vi "TAT_Varient Creater.vi"(8 "error in (no error)":errorcluster) -> (0 "error out":errorcluster)   [LabVIEW 2017]
uses:
  <vilib>/Utility/miscctls.llb/LVRangeTypeDef.ctl
  <vilib>/addons/database/Connection.llb/Conn ObjectReference.ctl
  <vilib>/Utility/miscctls.llb/LVRowAndColumnUnsignedTypeDef.ctl
  b1939813-2d0c-4b6e-8ee7-2e1edd5edc28.vi
  <vilib>/Utility/config.llb/Read Key (I32).vi
  <vilib>/Utility/config.llb/Read Key (String).vi
  <vilib>/Utility/config.llb/Write Key (U32).vi
  <vilib>/Utility/config.llb/Write Key (String).vi
  <vilib>/Utility/config.llb/NI_LVConfig.lvlib
  <vilib>/addons/database/NI_Database_API.lvlib
panel:
  in  "Vertical Slider Control":dbl(slide)=1.0
  in  "CANCLE 3":bool
  in  "PRINTING":bool
  in  "Manual print":bool
  in  "Cancle 2":bool
  in  "Delete Button":bool
  in  "Cancle":bool
  in  "Save Button":bool
  in  "TORISHI CODE":string
  in  "PART NUMBER":string
  in  "Delete Square":bool
  in  "EDIT & SAVE":bool
  out "Varient Details":string[][](table)
  in  "BATCH SIZE":u16=1 min=1 max=100 step=1
  in  "VARIENT NUMBER":u16=1 min=1 max=100 step=1
  in  "HOME":bool
  in  "UPDATE TABLE":bool
  in  "PART NAME":string(combo)
  # "Varient Creater"
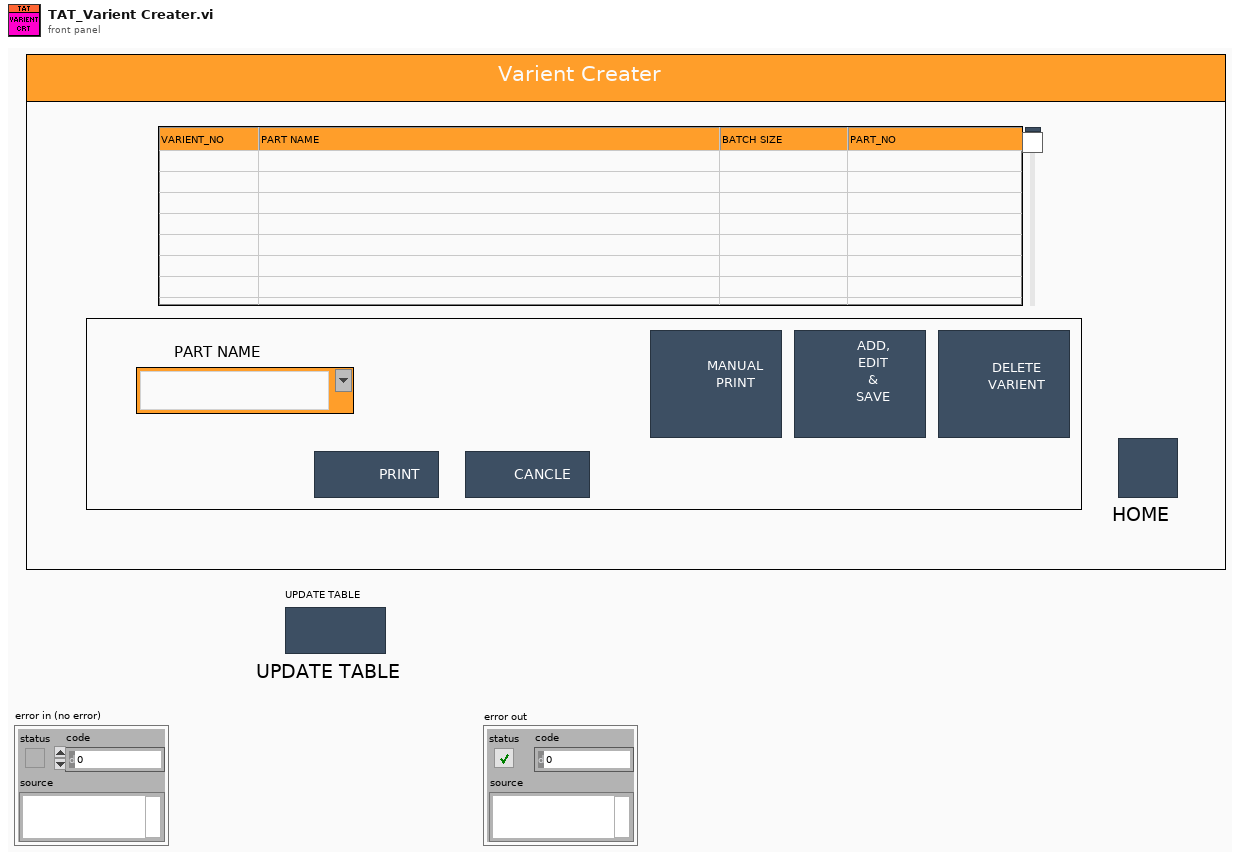
[diagram p1: front panel]
types:
  T1 = enum8{"Enabled", "Disabled", "Disabled and Grayed Out"}
  T2 = enum32{"invalid app kind", "Development System", "Run Time System", "Student Edition", "Embedded LabVIEW", "Evaluation", "Custom"}
  T3 = typedef "NI_LVConfig.lvlib/Config Data RefNum.ctl" = refnum<k1>
  T4 = typedef "LVRangeTypeDef.ctl" = cluster{"Minimum":dbl, "Maximum":dbl, "Increment":dbl, "Minor Increment":dbl, "Start":dbl}
  T5 = typedef "NI_Database_API.lvlib/Conn ObjectReference.ctl" = refnum<k1>
  T6 = cluster{"Varient number":u16, "Part name":string, "Barcode":string, "connection reference":T5, "Batch_Size":u16, "PART_NO":string, "TORISHI_CODE":string, "scanner com":refnum<visa-resource-name>, "Part Name List":string[], "Varient path":path, "Current Varient path":path, "Communication path":path, "PRN path":path, "printer":refnum<k5>, "Data_log_Path":path, "PREVIOUS Code":string[], "printer ip add":string}
  T7 = typedef "LVRowAndColumnUnsignedTypeDef.ctl" = cluster{"Row":u32, "Column":u32}
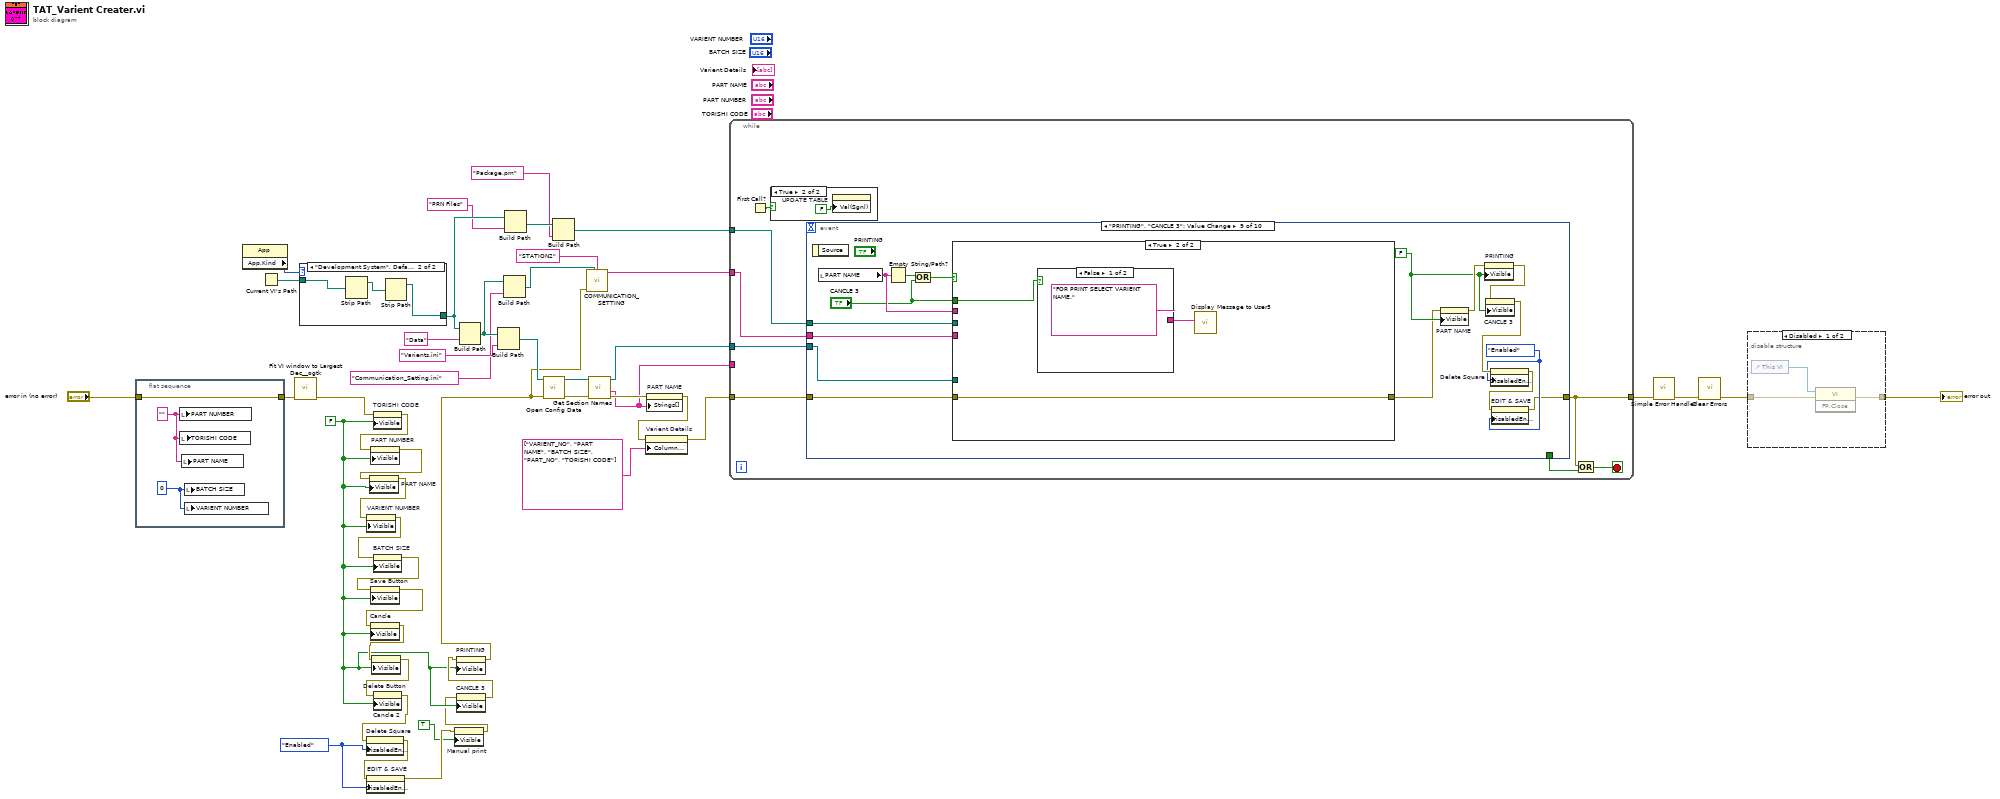
[diagram p0: block diagram]
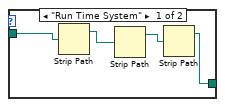
[diagram p3: hidden frame]
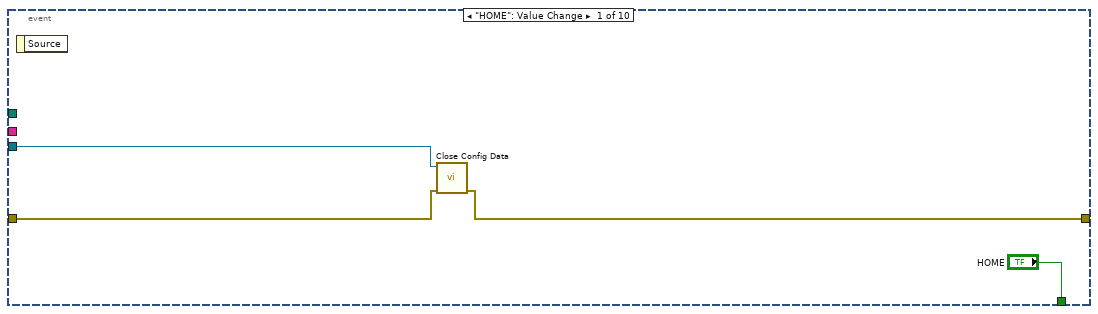
[diagram p5: hidden frame]
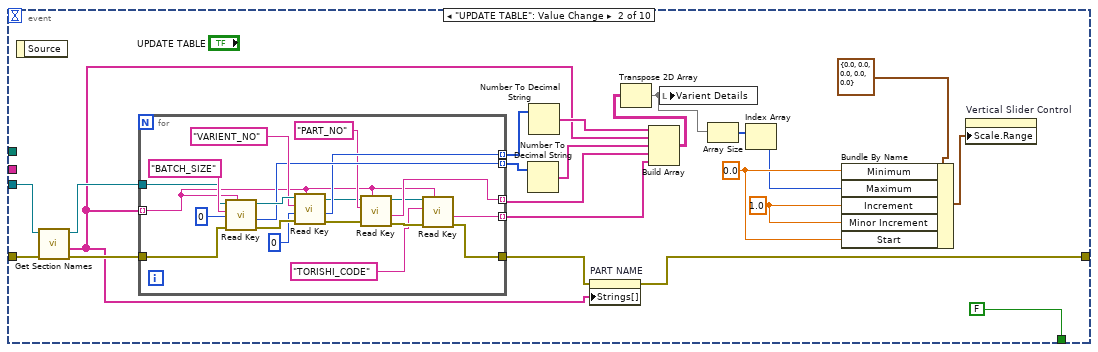
[diagram p6: hidden frame]
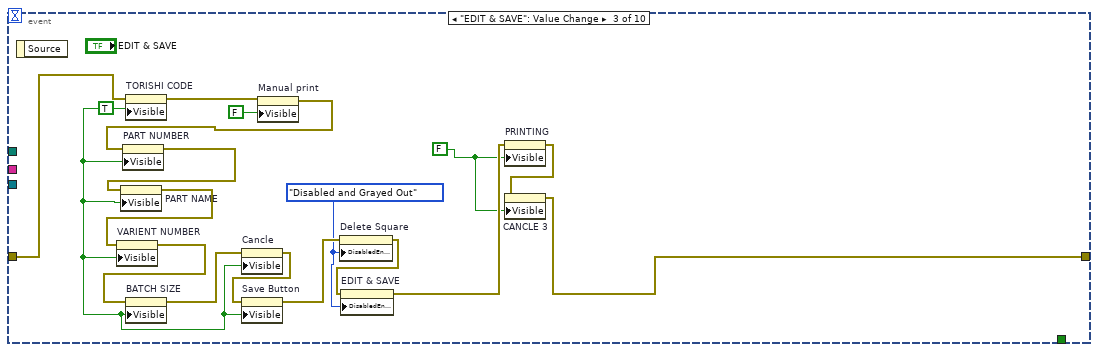
[diagram p7: hidden frame]
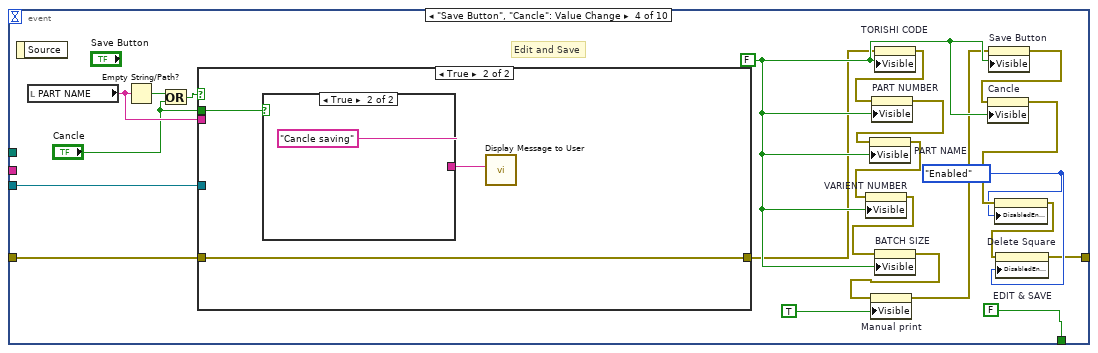
[diagram p8: hidden frame]
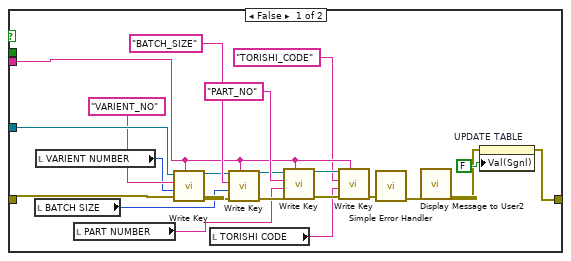
[diagram p9: hidden frame]
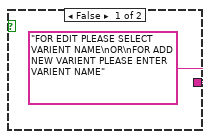
[diagram p10: hidden frame]
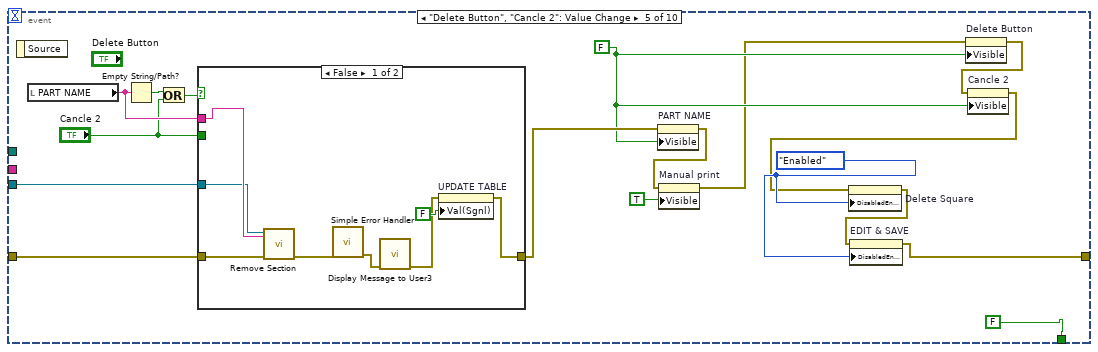
[diagram p11: hidden frame]
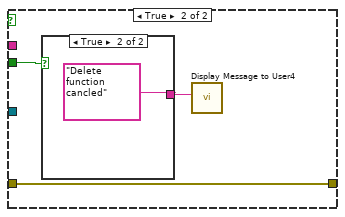
[diagram p12: hidden frame]
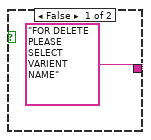
[diagram p13: hidden frame]
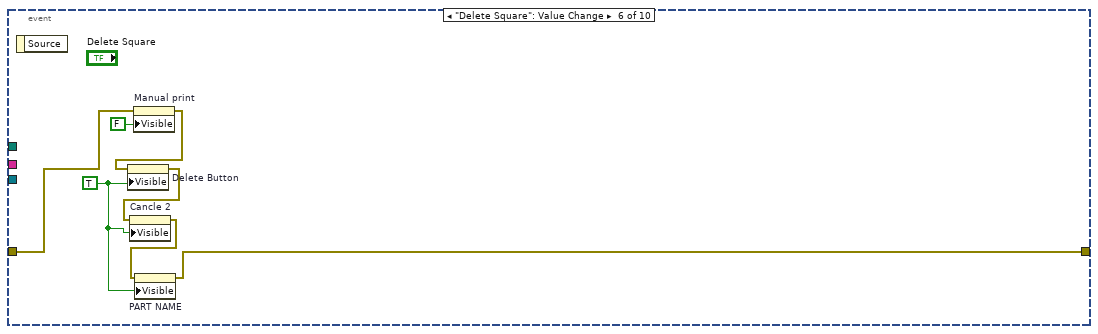
[diagram p14: hidden frame]
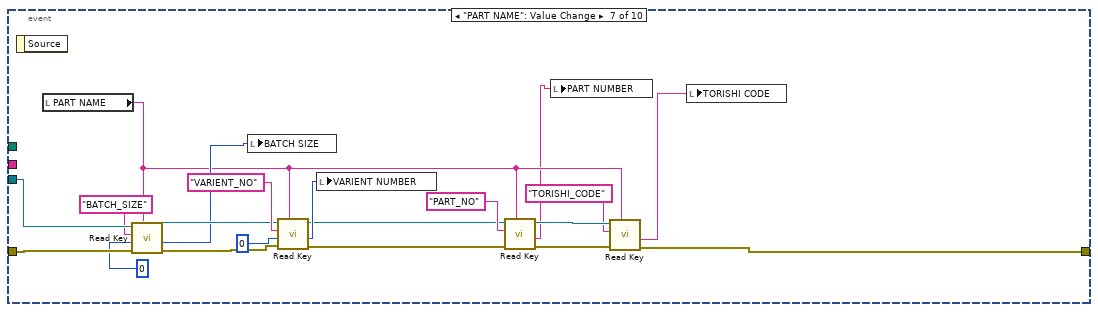
[diagram p15: hidden frame]
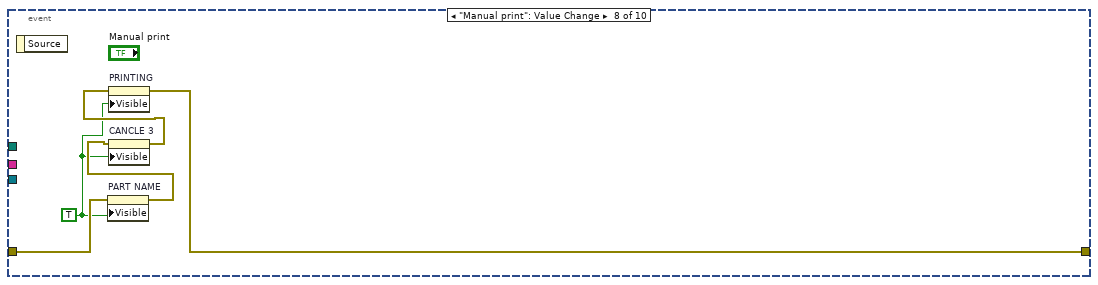
[diagram p16: hidden frame]
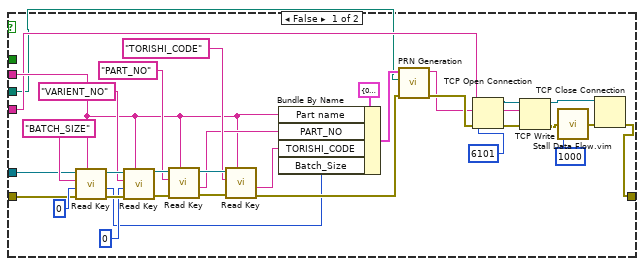
[diagram p17: hidden frame]
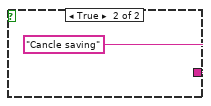
[diagram p18: hidden frame]
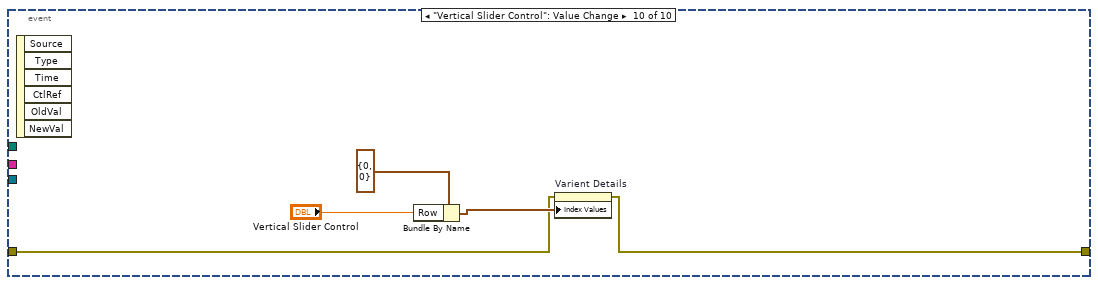
[diagram p19: hidden frame]
diagram:
  w21 = T1."Enabled" ("Disabled")
  w15 = FALSE
  n1 = flat-sequence {
    tunnel: [w48] -> w29
    tunnel: "error in (no error)" -> [w48]
    frame #0 {
      w49 = u16 0 ("BATCH SIZE")
      w50 = "" ("PART NUMBER")
      n2 = local write "PART NUMBER"(w50) -> ()
      n3 = local write "TORISHI CODE"(w50) -> ()
      n4 = local write "PART NAME"(w50) -> ()
      n5 = local write "BATCH SIZE"(w49) -> ()
      n6 = local write "VARIENT NUMBER"(w49) -> ()
    }
  }
  n7 = property class="App"() -> ("App.Kind"=w42:T2)  [unwired: 2 in, 2 out]
  n8 = Current VI's Path() -> (path=w43:path)
  n9 = call <userlib>:"Fit VI window to Largest Dec__ogtk.vi"("error in (no error)"=w29) -> ("error out"=w24:errorcluster)  [unwired: 5 in, 1 out]
  n10 = case shown="\"Development System\", Default" w42 {
    tunnel: w43 -> [w52 w56]
    tunnel: [w51 w55] -> w5
    frame "Run Time System" {
      n11 = Strip Path(path=w52) -> (stripped path=w54:path)  [unwired: 1 out]
      n12 = Strip Path(path=w54) -> (stripped path=w53:path)  [unwired: 1 out]
      n13 = Strip Path(path=w53) -> (stripped path=w51:path)  [unwired: 1 out]
    }
    frame "Development System", Default {
      n14 = Strip Path(path=w56) -> (stripped path=w57:path)  [unwired: 1 out]
      n15 = Strip Path(path=w57) -> (stripped path=w55:path)  [unwired: 1 out]
    }
  }
  n16 = property on="TORISHI CODE" class="Str"(error in=w24, "Visible"=w15) -> (error out=w28:errorcluster)  [unwired: 1 in, 1 out]
  n17 = property on="PART NUMBER" class="Str"(error in=w28, "Visible"=w15) -> (error out=w27:errorcluster)  [unwired: 1 in, 1 out]
  n18 = property on="PART NAME" class="CmbBox"(error in=w27, "Visible"=w15) -> (error out=w26:errorcluster)  [unwired: 1 in, 1 out]
  n19 = property on="VARIENT NUMBER" class="DigNum (strict)"(error in=w26, "Visible"=w15) -> (error out=w25:errorcluster)  [unwired: 1 in, 1 out]
  n20 = property on="BATCH SIZE" class="DigNum (strict)"(error in=w25, "Visible"=w15) -> (error out=w23:errorcluster)  [unwired: 1 in, 1 out]
  n21 = property on="Save Button" class="Bool"(error in=w23, "Visible"=w15) -> (error out=w20:errorcluster)  [unwired: 1 in, 1 out]
  n22 = property on="Cancle" class="Bool"(error in=w20, "Visible"=w15) -> (error out=w19:errorcluster)  [unwired: 1 in, 1 out]
  n23 = property on="Delete Button" class="Bool"(error in=w19, "Visible"=w15) -> (error out=w18:errorcluster)  [unwired: 1 in, 1 out]
  n24 = property on="Cancle 2" class="Bool"(error in=w18, "Visible"=w15) -> (error out=w17:errorcluster)  [unwired: 1 in, 1 out]
  n25 = property on="Delete Square" class="Bool"(error in=w17, "DisabledEnum"=w21) -> (error out=w22:errorcluster)  [unwired: 1 in, 1 out]
  n26 = property on="EDIT & SAVE" class="Bool"(error in=w22, "DisabledEnum"=w21) -> (error out=w14:errorcluster)  [unwired: 1 in, 1 out]
  n27 = property on="Manual print" class="Bool"(error in=w14, "Visible"=TRUE) -> (error out=w13:errorcluster)  [unwired: 1 in, 1 out]
  n28 = property on="CANCLE 3" class="Bool"(error in=w13, "Visible"=w15) -> (error out=w16:errorcluster)  [unwired: 1 in, 1 out]
  n29 = property on="PRINTING" class="Bool"(error in=w16, "Visible"=w15) -> (error out=w7:errorcluster)  [unwired: 1 in, 1 out]
  n30 = Build Path(base path=w5, name or relative path="Data") -> (appended path=w11:path)
  n31 = Build Path(base path=w11, name or relative path="Varients.ini") -> (appended path=w41:path)
  n32 = Build Path(base path=w11, name or relative path="Communication_Setting.ini") -> (appended path=w8:path)
  n33 = Build Path(base path=w5, name or relative path="PRN Files") -> (appended path=w3:path)
  n34 = call <vilib>:"Open Config Data.vi"("error in (no error)"=w7, "configuration file path"=w41) -> ("error out"=w37:errorcluster, "refnum"=w38:T3)  [unwired: 7 in, 1 out]
  n35 = Build Path(base path=w3, name or relative path="Package.prn") -> (appended path=w1:path)
  n36 = call "COMMUNICATION_SETTING.vi"("communication path"=w8, "error in"=w7, "STATION"="STATION2") -> ("PRINT_COM"=w6:string)  [unwired: 6 in, 2 out]
  n37 = call <vilib>:"Get Section Names.vi"("error in (no error)"=w37, "refnum"=w38) -> ("error out"=w36:errorcluster, "section names"=w31:string[], "refnum out"=w35:T3)  [unwired: 7 in]
  n38 = property on="PART NAME" class="CmbBox"(error in=w36, "Strings[]"=w31) -> (error out=w34:errorcluster)  [unwired: 1 in, 1 out]
  n39 = property on="Varient Details" class="Tbl (strict)"(error in=w34, "Column Headers[]"=string[] ["VARIENT_NO", "PART NAME", "BATCH SIZE", "PART_NO", "TORISHI CODE"] ("Column Header Strings[]")) -> (error out=w33:errorcluster)  [unwired: 1 in, 1 out]
  n40 = while {
    tunnel: w33 -> [w64]
    tunnel: [w62] -> w44
    tunnel: w35 -> [w61]
    tunnel: w31 -> [_]
    tunnel: w6 -> [w59]
    tunnel: w1 -> [w58]
    stop <- w63 stop-if-true
    n41 = First Call?() -> (First Call?: T/F=w60:bool)
    n42 = case shown="True" w60 {
      frame False {
      }
      frame True {
        n43 = property on="UPDATE TABLE" class="Bool (strict)"("Val(Sgnl)"=FALSE) -> ()  [unwired: 2 in, 2 out]
      }
    }
    n44 = event shown="[8] \"PRINTING\", \"CANCLE 3\": Value Change" {
      selector: _ -> [_ _ _ _ _ _ _ _ _ _]
      dyn-events: _ -> [_ _ _ _ _ _ _ _ _ _]
      timeout: _ -> [_ _ _ _ _ _ _ _ _ _]
      tunnel: ["HOME" FALSE ("stop") _ FALSE ("stop") FALSE ("stop") _ _ _ _ _] -> w65
      tunnel: w64 -> [w69 w86 w126 w148 w192 w209 w234 w237 w255 w294]
      tunnel: [w68 w78 w114 w133 w184 w212 w221 w236 w244 w295] -> w62
      tunnel: w61 -> [w67 w84 _ w149 w193 _ w233 _ w251 _]
      tunnel: w59 -> [_ _ _ _ _ _ _ _ w242 _]
      tunnel: w58 -> [_ _ _ _ _ _ _ _ w241 _]
      event "HOME": Value Change {
        n45 = event-data() -> ()  [unwired: 1 in, 1 out]
        n46 = call <vilib>:"Close Config Data.vi"("error in (no error)"=w69, "refnum"=w67) -> ("error out"=w68:errorcluster)  [unwired: 8 in, 1 out]
      }
      event "UPDATE TABLE": Value Change {
        w75 = 1.0 ("Increment")
        w74 = 0.0 ("Minimum")
        n47 = event-data() -> ()  [unwired: 1 in, 1 out]
        n48 = call <vilib>:"Get Section Names.vi"("error in (no error)"=w86, "refnum"=w84) -> ("error out"=w85:errorcluster, "section names"=w79:string[], "refnum out"=w83:T3)  [unwired: 7 in]
        n49 = for {
          tunnel: [w97] -> w80
          tunnel: w85 -> [w106]
          tunnel: w79 -> [w94] mode=indexing
          tunnel: w83 -> [w105]
          tunnel: [w104] -> w90 mode=indexing
          tunnel: [w103] -> w91 mode=indexing
          tunnel: [w99] -> w82 mode=indexing
          tunnel: [w93] -> w81 mode=indexing
          n50 = call-poly <vilib>:"Read Key.vi"("section"=w94, "error in (no error)"=w106, "default value"=0, "key"="BATCH_SIZE", "refnum"=w105) -> ("error out"=w112:errorcluster, "value"=w104:i32, "refnum out"=w111:T3)  [unwired: 3 in, 1 out]
          n51 = call-poly <vilib>:"Read Key.vi"("section"=w94, "error in (no error)"=w112, "default value"=0, "key"="VARIENT_NO", "refnum"=w111) -> ("error out"=w102:errorcluster, "value"=w103:i32, "refnum out"=w100:T3)  [unwired: 3 in, 1 out]
          n52 = call-poly <vilib>:"Read Key.vi"("section"=w94, "error in (no error)"=w102, "key"="PART_NO", "refnum"=w100) -> ("error out"=w98:errorcluster, "value"=w99:string, "refnum out"=w96:T3)  [unwired: 4 in, 1 out]
          n53 = call-poly <vilib>:"Read Key.vi"("section"=w94, "error in (no error)"=w98, "key"="TORISHI_CODE", "refnum"=w96) -> ("error out"=w97:errorcluster, "value"=w93:string)  [unwired: 4 in, 2 out]
        }
        n54 = Number To Decimal String(number=w90) -> (decimal integer string=w89:string[])  [unwired: 1 in]
        n55 = Number To Decimal String(number=w91) -> (decimal integer string=w87:string[])  [unwired: 1 in]
        n56 = property on="PART NAME" class="CmbBox"(error in=w80, "Strings[]"=w79) -> (error out=w78:errorcluster)  [unwired: 1 in, 1 out]
        n57 = Build Array(w87, w79, w89, w82, w81) -> (w88:string[][])
        n58 = Transpose 2D Array(2D array=w88) -> (transposed array=w77:string[][])
        n59 = local write "Varient Details"(w77) -> ()
        n60 = Array Size(array=w77) -> (size(s)=w76:i32[])
        n61 = Index Array(array=w76) -> (element=w71:i32)  [unwired: 1 in]
        n62 = Bundle By Name(cluster=T4 {"Minimum"=0.0, "Maximum"=0.0, "Increment"=0.0, "Minor Increment"=0.0, "Start"=0.0} ("Scale.Range"), "Minimum"=w74, "Maximum"=w71, "Increment"=w75, "Minor Increment"=w75, "Start"=w74) -> (w73:T4)
        n63 = property on="Vertical Slider Control" class="Slide (strict)"("Scale.Range"=w73) -> ()  [unwired: 2 in, 2 out]
      }
      event "EDIT & SAVE": Value Change {
        w113 = FALSE
        w123 = T1."Disabled and Grayed Out" ("Disabled")
        w120 = TRUE
        n64 = event-data() -> ()  [unwired: 1 in, 1 out]
        n65 = property on="TORISHI CODE" class="Str"(error in=w126, "Visible"=w120) -> (error out=w119:errorcluster)  [unwired: 1 in, 1 out]
        n66 = property on="Manual print" class="Bool"(error in=w119, "Visible"=FALSE) -> (error out=w118:errorcluster)  [unwired: 1 in, 1 out]
        n67 = property on="PART NUMBER" class="Str"(error in=w118, "Visible"=w120) -> (error out=w127:errorcluster)  [unwired: 1 in, 1 out]
        n68 = property on="PART NAME" class="CmbBox"(error in=w127, "Visible"=w120) -> (error out=w128:errorcluster)  [unwired: 1 in, 1 out]
        n69 = property on="VARIENT NUMBER" class="DigNum (strict)"(error in=w128, "Visible"=w120) -> (error out=w129:errorcluster)  [unwired: 1 in, 1 out]
        n70 = property on="BATCH SIZE" class="DigNum (strict)"(error in=w129, "Visible"=w120) -> (error out=w121:errorcluster)  [unwired: 1 in, 1 out]
        n71 = property on="Cancle" class="Bool"(error in=w121, "Visible"=w120) -> (error out=w122:errorcluster)  [unwired: 1 in, 1 out]
        n72 = property on="Save Button" class="Bool"(error in=w122, "Visible"=w120) -> (error out=w125:errorcluster)  [unwired: 1 in, 1 out]
        n73 = property on="Delete Square" class="Bool"(error in=w125, "DisabledEnum"=w123) -> (error out=w124:errorcluster)  [unwired: 1 in, 1 out]
        n74 = property on="EDIT & SAVE" class="Bool"(error in=w124, "DisabledEnum"=w123) -> (error out=w115:errorcluster)  [unwired: 1 in, 1 out]
        n75 = property on="PRINTING" class="Bool"(error in=w115, "Visible"=w113) -> (error out=w116:errorcluster)  [unwired: 1 in, 1 out]
        n76 = property on="CANCLE 3" class="Bool"(error in=w116, "Visible"=w113) -> (error out=w114:errorcluster)  [unwired: 1 in, 1 out]
      }
      event "Save Button", "Cancle": Value Change {
        w135 = T1."Enabled" ("Disabled")
        w136 = FALSE
        # "Edit and Save"
        n77 = event-data() -> ()  [unwired: 1 in, 1 out]
        n78 = local read "PART NAME"() -> (w147:string)
        n79 = Empty String/Path?(string/path=w147) -> (empty?=w146:bool)
        n80 = Or(x=w146, y="Cancle") -> (x .or. y?=w145:bool)
        n81 = case shown="True" w145 {
          tunnel: w148 -> [w171 w175]
          tunnel: [w165 w175] -> w134
          tunnel: w149 -> [w169 _]
          tunnel: w147 -> [w154 _]
          tunnel: "Cancle" -> [_ w173]
          frame False {
            n82 = local read "BATCH SIZE"() -> (w164:u16)
            n83 = local read "VARIENT NUMBER"() -> (w163:u16)
            n84 = local read "PART NUMBER"() -> (w151:string)
            n85 = call-poly <vilib>:"Write Key.vi"("section"=w154, "error in (no error)"=w171, "value"=w163, "key"="VARIENT_NO", "refnum"=w169) -> ("error out"=w170:errorcluster, "refnum out"=w168:T3)  [unwired: 4 in, 1 out]
            n86 = local read "TORISHI CODE"() -> (w152:string)
            n87 = call-poly <vilib>:"Write Key.vi"("section"=w154, "error in (no error)"=w170, "value"=w164, "key"="BATCH_SIZE", "refnum"=w168) -> ("error out"=w158:errorcluster, "refnum out"=w155:T3)  [unwired: 4 in, 1 out]
            n88 = call-poly <vilib>:"Write Key.vi"("section"=w154, "error in (no error)"=w158, "value"=w151, "key"="PART_NO", "refnum"=w155) -> ("error out"=w159:errorcluster, "refnum out"=w160:T3)  [unwired: 4 in, 1 out]
            n89 = call-poly <vilib>:"Write Key.vi"("section"=w154, "error in (no error)"=w159, "value"=w152, "key"="TORISHI_CODE", "refnum"=w160) -> ("error out"=w157:errorcluster)  [unwired: 4 in, 2 out]
            n90 = call <vilib>:"Simple Error Handler.vi"("error in (no error)"=w157) -> ("error out"=w162:errorcluster)  [unwired: 4 in, 4 out]
            n91 = call "Display Message to User2"("error in (no error)"=w162) -> ("error out"=w161:errorcluster)  [unwired: 9 in, 1 out]
            n92 = property on="UPDATE TABLE" class="Bool (strict)"(error in=w161, "Val(Sgnl)"=FALSE) -> (error out=w165:errorcluster)  [unwired: 1 in, 1 out]
          }
          frame True {
            n93 = case shown="True" w173 {
              tunnel: ["FOR EDIT PLEASE SELECT VARIENT NAME\nOR\nFOR ADD NEW VARIENT PLEASE ENTER VARIENT NAME" "Cancle saving"] -> w174
              frame False {
              }
              frame True {
              }
            }
            n94 = call "Display Message to User"("Message"=w174) -> ()  [unwired: 9 in, 2 out]
          }
        }
        n95 = property on="TORISHI CODE" class="Str"(error in=w134, "Visible"=w136) -> (error out=w143:errorcluster)  [unwired: 1 in, 1 out]
        n96 = property on="PART NUMBER" class="Str"(error in=w143, "Visible"=w136) -> (error out=w142:errorcluster)  [unwired: 1 in, 1 out]
        n97 = property on="PART NAME" class="CmbBox"(error in=w142, "Visible"=w136) -> (error out=w141:errorcluster)  [unwired: 1 in, 1 out]
        n98 = property on="VARIENT NUMBER" class="DigNum (strict)"(error in=w141, "Visible"=w136) -> (error out=w140:errorcluster)  [unwired: 1 in, 1 out]
        n99 = property on="BATCH SIZE" class="DigNum (strict)"(error in=w140, "Visible"=w136) -> (error out=w131:errorcluster)  [unwired: 1 in, 1 out]
        n100 = property on="Manual print" class="Bool"(error in=w131, "Visible"=TRUE) -> (error out=w130:errorcluster)  [unwired: 1 in, 1 out]
        n101 = property on="Save Button" class="Bool"(error in=w130, "Visible"=w136) -> (error out=w138:errorcluster)  [unwired: 1 in, 1 out]
        n102 = property on="Cancle" class="Bool"(error in=w138, "Visible"=w136) -> (error out=w137:errorcluster)  [unwired: 1 in, 1 out]
        n103 = property on="Delete Square" class="Bool"(error in=w137, "DisabledEnum"=w135) -> (error out=w139:errorcluster)  [unwired: 1 in, 1 out]
        n104 = property on="EDIT & SAVE" class="Bool"(error in=w139, "DisabledEnum"=w135) -> (error out=w133:errorcluster)  [unwired: 1 in, 1 out]
      }
      event "Delete Button", "Cancle 2": Value Change {
        w186 = T1."Enabled" ("Disabled")
        w181 = FALSE
        n105 = event-data() -> ()  [unwired: 1 in, 1 out]
        n106 = local read "PART NAME"() -> (w191:string)
        n107 = Empty String/Path?(string/path=w191) -> (empty?=w190:bool)
        n108 = Or(x=w190, y="Cancle 2") -> (x .or. y?=w189:bool)
        n109 = case shown="False" w189 {
          tunnel: w192 -> [w196 w205]
          tunnel: [w201 w205] -> w185
          tunnel: w193 -> [w197 _]
          tunnel: w191 -> [w198 _]
          tunnel: "Cancle 2" -> [_ w204]
          frame False {
            n110 = call <vilib>:"Remove Section.vi"("section"=w198, "error in (no error)"=w196, "refnum"=w197) -> ("error out"=w195:errorcluster)  [unwired: 6 in, 2 out]
            n111 = call <vilib>:"Simple Error Handler.vi"("error in (no error)"=w195) -> ("error out"=w200:errorcluster)  [unwired: 4 in, 4 out]
            n112 = call "Display Message to User3"("error in (no error)"=w200) -> ("error out"=w199:errorcluster)  [unwired: 9 in, 1 out]
            n113 = property on="UPDATE TABLE" class="Bool (strict)"(error in=w199, "Val(Sgnl)"=FALSE) -> (error out=w201:errorcluster)  [unwired: 1 in, 1 out]
          }
          frame True {
            n114 = case shown="True" w204 {
              tunnel: ["FOR DELETE PLEASE SELECT VARIENT NAME" "Delete function cancled"] -> w203
              frame False {
              }
              frame True {
              }
            }
            n115 = call "Display Message to User4"("Message"=w203) -> ()  [unwired: 9 in, 2 out]
          }
        }
        n116 = property on="PART NAME" class="CmbBox"(error in=w185, "Visible"=w181) -> (error out=w179:errorcluster)  [unwired: 1 in, 1 out]
        n117 = property on="Manual print" class="Bool"(error in=w179, "Visible"=TRUE) -> (error out=w178:errorcluster)  [unwired: 1 in, 1 out]
        n118 = property on="Delete Button" class="Bool"(error in=w178, "Visible"=w181) -> (error out=w183:errorcluster)  [unwired: 1 in, 1 out]
        n119 = property on="Cancle 2" class="Bool"(error in=w183, "Visible"=w181) -> (error out=w182:errorcluster)  [unwired: 1 in, 1 out]
        n120 = property on="Delete Square" class="Bool"(error in=w182, "DisabledEnum"=w186) -> (error out=w187:errorcluster)  [unwired: 1 in, 1 out]
        n121 = property on="EDIT & SAVE" class="Bool"(error in=w187, "DisabledEnum"=w186) -> (error out=w184:errorcluster)  [unwired: 1 in, 1 out]
      }
      event "Delete Square": Value Change {
        w211 = TRUE
        n122 = event-data() -> ()  [unwired: 1 in, 1 out]
        n123 = property on="Manual print" class="Bool"(error in=w209, "Visible"=FALSE) -> (error out=w208:errorcluster)  [unwired: 1 in, 1 out]
        n124 = property on="Delete Button" class="Bool"(error in=w208, "Visible"=w211) -> (error out=w214:errorcluster)  [unwired: 1 in, 1 out]
        n125 = property on="Cancle 2" class="Bool"(error in=w214, "Visible"=w211) -> (error out=w213:errorcluster)  [unwired: 1 in, 1 out]
        n126 = property on="PART NAME" class="CmbBox"(error in=w213, "Visible"=w211) -> (error out=w212:errorcluster)  [unwired: 1 in, 1 out]
      }
      event "PART NAME": Value Change {
        n127 = event-data() -> ()  [unwired: 1 in, 1 out]
        n128 = local read "PART NAME"() -> (w217:string)
        n129 = call-poly <vilib>:"Read Key.vi"("section"=w217, "error in (no error)"=w234, "default value"=0, "key"="BATCH_SIZE", "refnum"=w233) -> ("error out"=w230:errorcluster, "value"=w225:i32, "refnum out"=w229:T3)  [unwired: 3 in, 1 out]
        n130 = local write "BATCH SIZE"(w225) -> ()
        n131 = call-poly <vilib>:"Read Key.vi"("section"=w217, "error in (no error)"=w230, "default value"=0, "key"="VARIENT_NO", "refnum"=w229) -> ("error out"=w222:errorcluster, "value"=w228:i32, "refnum out"=w218:T3)  [unwired: 3 in, 1 out]
        n132 = local write "VARIENT NUMBER"(w228) -> ()
        n133 = call-poly <vilib>:"Read Key.vi"("section"=w217, "error in (no error)"=w222, "key"="PART_NO", "refnum"=w218) -> ("error out"=w223:errorcluster, "value"=w216:string, "refnum out"=w224:T3)  [unwired: 4 in, 1 out]
        n134 = local write "PART NUMBER"(w216) -> ()
        n135 = call-poly <vilib>:"Read Key.vi"("section"=w217, "error in (no error)"=w223, "key"="TORISHI_CODE", "refnum"=w224) -> ("error out"=w221:errorcluster, "value"=w215:string)  [unwired: 4 in, 2 out]
        n136 = local write "TORISHI CODE"(w215) -> ()
      }
      event "Manual print": Value Change {
        w235 = TRUE
        n137 = event-data() -> ()  [unwired: 1 in, 1 out]
        n138 = property on="PART NAME" class="CmbBox"(error in=w237, "Visible"=w235) -> (error out=w239:errorcluster)  [unwired: 1 in, 1 out]
        n139 = property on="CANCLE 3" class="Bool"(error in=w239, "Visible"=w235) -> (error out=w238:errorcluster)  [unwired: 1 in, 1 out]
        n140 = property on="PRINTING" class="Bool"(error in=w238, "Visible"=w235) -> (error out=w236:errorcluster)  [unwired: 1 in, 1 out]
      }
      event "PRINTING", "CANCLE 3": Value Change {
        w245 = T1."Enabled" ("Disabled")
        w246 = FALSE
        n141 = event-data() -> ()  [unwired: 1 in, 1 out]
        n142 = local read "PART NAME"() -> (w252:string)
        n143 = Empty String/Path?(string/path=w252) -> (empty?=w254:bool)
        n144 = Or(x=w254, y="CANCLE 3") -> (x .or. y?=w253:bool)
        n145 = case shown="True" w253 {
          tunnel: w255 -> [w277 w291]
          tunnel: [w264 w291] -> w243
          tunnel: w252 -> [w258 _]
          tunnel: w251 -> [w276 _]
          tunnel: w242 -> [w257 _]
          tunnel: w241 -> [w256 _]
          tunnel: "CANCLE 3" -> [_ w289]
          frame False {
            n146 = call-poly <vilib>:"Read Key.vi"("section"=w258, "error in (no error)"=w277, "default value"=0, "key"="BATCH_SIZE", "refnum"=w276) -> ("error out"=w288:errorcluster, "value"=w261:i32, "refnum out"=w287:T3)  [unwired: 3 in, 1 out]
            n147 = call-poly <vilib>:"Read Key.vi"("section"=w258, "error in (no error)"=w288, "default value"=0, "key"="VARIENT_NO", "refnum"=w287) -> ("error out"=w284:errorcluster, "refnum out"=w283:T3)  [unwired: 3 in, 2 out]
            n148 = call-poly <vilib>:"Read Key.vi"("section"=w258, "error in (no error)"=w284, "key"="PART_NO", "refnum"=w283) -> ("error out"=w285:errorcluster, "value"=w259:string, "refnum out"=w286:T3)  [unwired: 4 in, 1 out]
            n149 = call-poly <vilib>:"Read Key.vi"("section"=w258, "error in (no error)"=w285, "key"="TORISHI_CODE", "refnum"=w286) -> ("error out"=w263:errorcluster, "value"=w262:string)  [unwired: 4 in, 2 out]
            n150 = Bundle By Name(cluster=T6 {"Varient number"=0, "Part name"="", "Barcode"="", "connection reference"=refnum, "Batch_Size"=0, "PART_NO"="", "TORISHI_CODE"="", "scanner com"="", "Part Name List"=[], "Varient path"=path "", "Current Varient path"=path "", "Communication path"=path "", "PRN path"=path "", "printer"=refnum, "Data_log_Path"=path "", "PREVIOUS Code"=[], "printer ip add"=""} ("Cluster"), "Part name"=w258, "PART_NO"=w259, "TORISHI_CODE"=w262, "Batch_Size"=w261) -> (w275:T6)
            n151 = call "PRN Generation.vi"("error in (no error)"=w263, "PRN path"=w256, "Cluster"=w275) -> ("error out"=w270:errorcluster, "PRN to Print"=w268:string)  [unwired: 7 in]
            n152 = TCP Open Connection(address=w257, remote port or service name=u16 6101, error in (no error)=w270) -> (connection ID=w272:refnum<k5>, error out=w271:errorcluster)  [unwired: 2 in]
            n153 = TCP Write(connection ID=w272, data in=w268, error in (no error)=w271) -> (connection ID out=w274:refnum<k5>, error out=w269:errorcluster)  [unwired: 1 in, 1 out]
            n154 = call "Stall Data Flow.vim"("value in"=w269, "milliseconds to wait"=u32 1000) -> ("value out"=w273:errorcluster)  [unwired: 1 out]
            n155 = TCP Close Connection(connection ID=w274, error in (no error)=w273) -> (error out=w264:errorcluster)  [unwired: 1 in, 1 out]
          }
          frame True {
            n156 = case shown="False" w289 {
              tunnel: ["FOR PRINT SELECT VARIENT NAME." "Cancle saving"] -> w290
              frame False {
              }
              frame True {
              }
            }
            n157 = call "Display Message to User5"("Message"=w290) -> ()  [unwired: 9 in, 2 out]
          }
        }
        n158 = property on="PART NAME" class="CmbBox"(error in=w243, "Visible"=w246) -> (error out=w250:errorcluster)  [unwired: 1 in, 1 out]
        n159 = property on="PRINTING" class="Bool"(error in=w250, "Visible"=w246) -> (error out=w248:errorcluster)  [unwired: 1 in, 1 out]
        n160 = property on="CANCLE 3" class="Bool"(error in=w248, "Visible"=w246) -> (error out=w247:errorcluster)  [unwired: 1 in, 1 out]
        n161 = property on="Delete Square" class="Bool"(error in=w247, "DisabledEnum"=w245) -> (error out=w249:errorcluster)  [unwired: 1 in, 1 out]
        n162 = property on="EDIT & SAVE" class="Bool"(error in=w249, "DisabledEnum"=w245) -> (error out=w244:errorcluster)  [unwired: 1 in, 1 out]
      }
      event "Vertical Slider Control": Value Change {
        n163 = event-data() -> ()  [unwired: 1 in, 6 out]
        n164 = Bundle By Name(cluster=T7 {"Row"=0, "Column"=0} ("Index Values"), "Row"="Vertical Slider Control") -> (w297:T7)
        n165 = property on="Varient Details" class="Tbl (strict)"(error in=w294, "Index Values"=w297) -> (error out=w295:errorcluster)  [unwired: 1 in, 1 out]
      }
    }
    n166 = Or(x=w62, y=w65) -> (x .or. y?=w63:bool)
  }
  n167 = call <vilib>:"Simple Error Handler.vi"("error in (no error)"=w44) -> ("error out"=w47:errorcluster)  [unwired: 4 in, 4 out]
  n168 = call <vilib>:"Clear Errors.vi"("error in (no error)"=w47) -> ("error out"=w46:errorcluster)  [unwired: 5 in, 1 out]
  n169 = disable-structure shown="Disabled" {
    disable-tunnel: w46 -> [w301 w302]
    disable-tunnel: [w300 w302] -> w45
    frame Disabled {
      n170 = control-ref of="This VI"() -> (w299:refnum<vi>)
      n171 = invoke class="VI" method="FP.Close"(reference=w299, error in=w301) -> (error out=w300:errorcluster)  [unwired: 1 in, 2 out]
    }
    frame Enabled {
    }
  }
  "error out" <- w45
